vi "versnelling (SubVI).vi"(8 "snelheid van de motor rechts":dbl, 9 "snelheid van de motor links":dbl, 10 "afstandssensor":dbl, 11 "OK Button":bool) -> (0 "snelheid van de motor rechts   2":dbl, 1 "snelheid van de motor links   2":dbl)   [LabVIEW 2019]
uses:
  <vilib>/myRIO/Express VI/Onboard IO/PWM/PWM Express VI.xnode
  <vilib>/myRIO/Instrument Drivers/Onboard IO/PWM/vis/Set Duty Cycle and Frequency.vi
  <vilib>/myRIO/Instrument Drivers/Onboard IO/PWM/PWM.lvlib
  <vilib>/myRIO/Instrument Drivers/Onboard IO/PWM/typedefs/PWM Configuration.ctl
  <vilib>/myRIO/Common/Instrument Driver Framework/myRIO v1.0/PWM/typedefs/PWM Channels Enum.ctl
  <vilib>/myRIO/Common/Instrument Driver Framework/Utilities/typedefs/Generic FPGA Reference.ctl
  <vilib>/myRIO/Common/Instrument Driver Framework/Utilities/typedefs/myRIO v1.0 Reference.ctl
  <vilib>/myRIO/Common/Instrument Driver Framework/Utilities/typedefs/Hardware Version Enum.ctl
  <vilib>/myRIO/Common/Instrument Driver Framework/Utilities/typedefs/myRIO Generic Hardware Reference.ctl
  <vilib>/myRIO/Instrument Drivers/Onboard IO/PWM/typedefs/PWM Reference.ctl
  <vilib>/myRIO/Instrument Drivers/Onboard IO/PWM/vis/myRIO PWM Open.xnode
  <vilib>/myRIO/Common/Instrument Driver Framework/Utilities/vis/Is FPGA Ref Available.vi
  <vilib>/myRIO/Common/Instrument Driver Framework/myRIO v1.0/PWM/vis/myRIO v1.1 Open PWM.vi
  <vilib>/userDefined/High Color/nirio_resource_hc.ctl
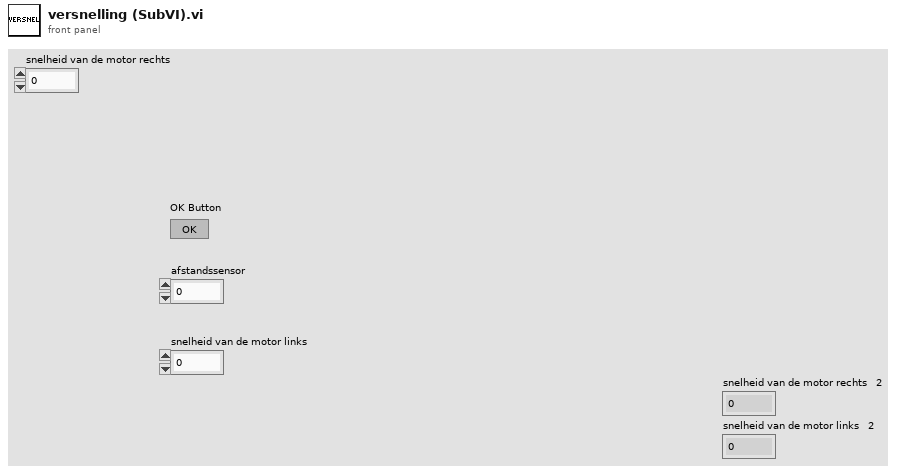
[diagram p1: front panel]
types:
  T1 = typedef "PWM.lvlib/PWM Reference.ctl" = cluster{"myRIO Reference":T2, "PWM Channels Enum":T6, "PWM Configuration":T7}
  T2 = typedef "myRIO Generic Hardware Reference.ctl" = cluster{"myRIO Model":T3, "myRIO Hardware Reference":T4}
  T3 = typedef "Hardware Version Enum.ctl" = enum16{"Unknown", "myRIO-1900", "myRIO-1950", "roboRIO", "NI ELVIS RIO CM", "ELVIS III"}
  T4 = typedef "myRIO v1.0 Reference.ctl" = cluster{"Generic FPGA Reference":T5, "Allow multiple opens":bool}
  T5 = typedef "Generic FPGA Reference.ctl" = refnum<k20>
  T6 = typedef "PWM Channels Enum.ctl" = enum16{"Not Connected", "C/PWM0", "C/PWM1", "A/PWM0", "A/PWM1", "A/PWM2", "A/PWM3", "A/PWM4", "A/PWM5", "A/PWM6", "A/PWM7", "A/PWM8", "A/PWM9", "A/PWM10", "A/PWM11", "A/PWM12", "A/PWM13", "A/PWM14", "A/PWM15", "A/PWM16", "A/PWM17", "A/PWM18", "A/PWM19", "B/PWM0", "B/PWM1", "B/PWM2", "B/PWM3", "B/PWM4", "B/PWM5", "B/PWM6", "B/PWM7", "B/PWM8", "B/PWM9", "B/PWM10", "B/PWM11", "B/PWM12", "B/PWM13", "B/PWM14", "B/PWM15", "B/PWM16", "B/PWM17", "B/PWM18", "B/PWM19", "PWM/PWM0", "PWM/PWM1", "PWM/PWM2", "PWM/PWM3", "PWM/PWM4", "PWM/PWM5", "PWM/PWM6", "PWM/PWM7", "PWM/PWM8", "PWM/PWM9"}
  T7 = typedef "PWM.lvlib/PWM Configuration.ctl" = cluster{"Frequency":dbl, "Duty Cycle":dbl}
  T8 = typedef "nirio_resource_hc.ctl" = tag
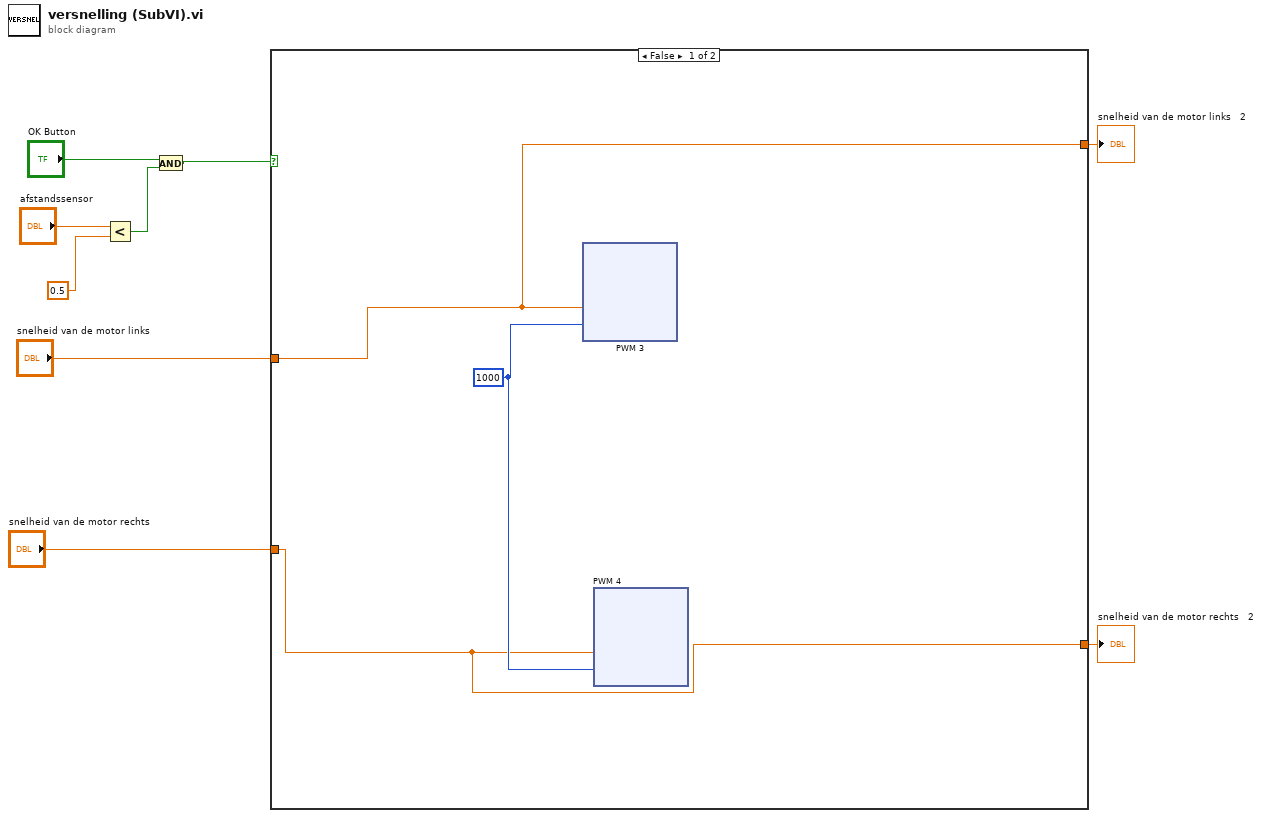
[diagram p0: block diagram]
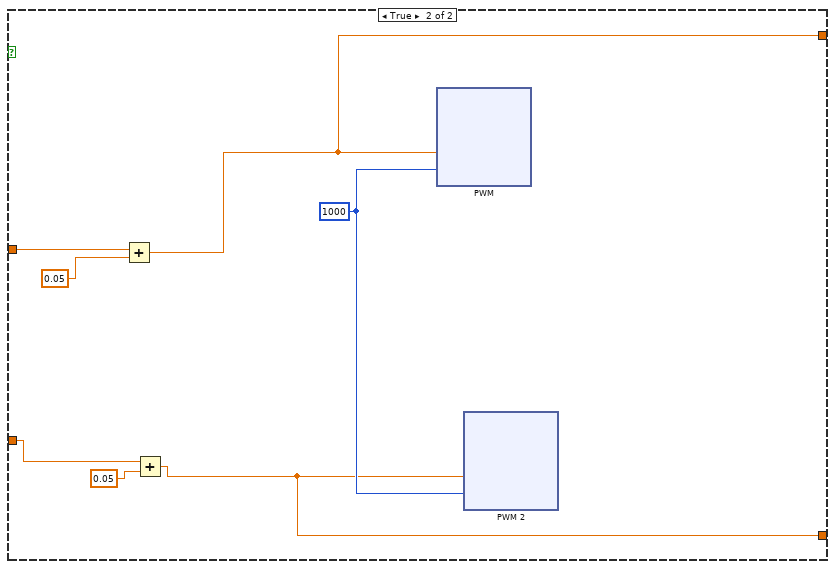
[diagram p2: hidden frame]
diagram:
  n1 = Less?(x="afstandssensor", y=0.5) -> (x < y?=w6:bool)
  n2 = And(x="OK Button", y=w6) -> (x .and. y?=w5:bool)
  n3 = case shown="False" w5 {
    tunnel: "snelheid van de motor links" -> [w11 w88]
    tunnel: "snelheid van de motor rechts" -> [w10 w85]
    tunnel: [w11 w84] -> w1
    tunnel: [w10 w83] -> w2
    frame False {
      w12 = 1000
      n4 = xnode "PWM 3"("Duty Cycle"=w11, "Frequency [Hz]"=w12) -> ()  [unwired: 1 in, 1 out]
      n5 = xnode "PWM 4"("Duty Cycle"=w10, "Frequency [Hz]"=w12) -> ()  [unwired: 1 in, 1 out]
    }
    frame True {
      w87 = 1000
      n6 = Add(x=w88, y=0.05) -> (x+y=w84:dbl)
      n7 = Add(x=w85, y=0.05) -> (x+y=w83:dbl)
      n8 = xnode "PWM"("Duty Cycle"=w84, "Frequency [Hz]"=w87) -> ()  [unwired: 1 in, 1 out]
      n9 = xnode "PWM 2"("Duty Cycle"=w83, "Frequency [Hz]"=w87) -> ()  [unwired: 1 in, 1 out]
    }
  }
  "snelheid van de motor rechts   2" <- w2
  "snelheid van de motor links   2" <- w1
